vi "Set Attributes To Ini File.vi"(8 "error in (no error)":errorcluster, 10 "Selection Name":string, 11 "UIConfiguration in":refnum<class "UIConfiguration.lvclass">) -> (0 "error out":errorcluster, 3 "UIConfiguration out":refnum<class "UIConfiguration.lvclass">)   [LabVIEW 2015, in "UIConfiguration.lvclass"]
uses:
  UIConfiguration.lvclass
  UIConfiguration.lvclass/UIConfiguration.ctl
  <vilib>/Utility/config.llb/NI_LVConfig.lvlib
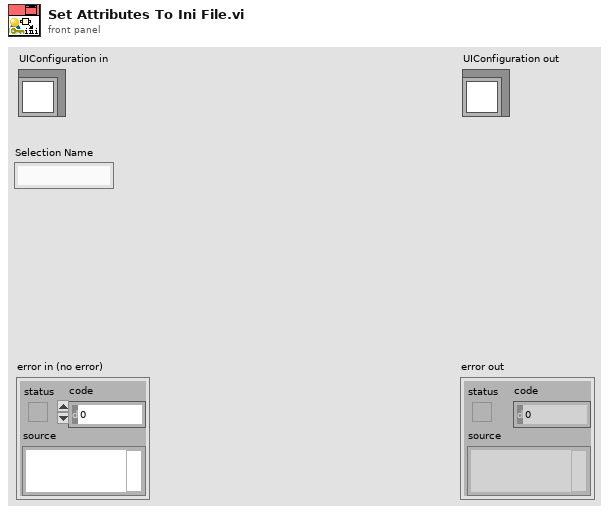
[diagram p1: front panel]
types:
  T1 = typedef "NI_LVConfig.lvlib/Config Data RefNum.ctl" = refnum<k1>
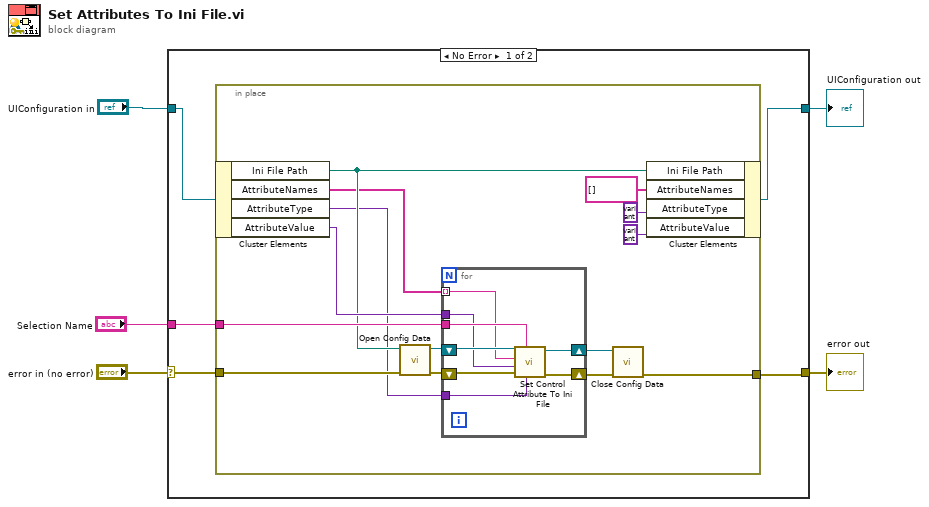
[diagram p0: block diagram]
diagram:
  n1 = case shown="No Error" "error in (no error)" {
    selector: "error in (no error)" -> [w9 w34]
    tunnel: [w7 w34] -> w4
    tunnel: [w6 w33] -> w2
    tunnel: "UIConfiguration in" -> [w10 w33]
    tunnel: "Selection Name" -> [w8 _]
    frame No Error {
      n2 = in-place {
        in-place-border: w9 -> [w24]
        in-place-border: w8 -> [w20]
        in-place-border: [w17] -> w7
        n3 = in-place-cluster #1(w10) -> ("Ini File Path"=w16:path, "AttributeNames"=w15:string[], "AttributeType"=w14:variant, "AttributeValue"=w21:variant)
        n4 = call <vilib>:"Open Config Data.vi"("error in (no error)"=w24, "configuration file path"=w16) -> ("error out"=w22:errorcluster, "refnum"=w23:T1)  [unwired: 7 in, 1 out]
        n5 = for {
          tunnel: w15 -> [w27] mode=indexing
          tunnel: w14 -> [w29]
          tunnel: w21 -> [w28]
          tunnel: w20 -> [w32]
          shift-right: [w26] -> w19
          shift-left: w23 -> [w31]
          shift-right: [w25] -> w18
          shift-left: w22 -> [w30]
          n6 = call "Set Control Attribute To Ini File.vi"("AttributeType"=w29, "Section"=w32, "error in (no error)"=w30, "AttributeValue"=w28, "AttributeNames"=w27, "INI Ref"=w31) -> ("error out"=w25:errorcluster, "Ini Ref out"=w26:T1)  [unwired: 4 in]
        }
        n7 = call <vilib>:"Close Config Data.vi"("error in (no error)"=w18, "refnum"=w19) -> ("error out"=w17:errorcluster)  [unwired: 8 in, 1 out]
        n8 = in-place-cluster #1("Ini File Path"=w16, "AttributeNames"=string[] [], "AttributeType"=variant, "AttributeValue"=variant) -> (w6:refnum<class "UIConfiguration.lvclass">)
      }
    }
    frame Error {
    }
  }
  "error out" <- w4
  "UIConfiguration out" <- w2
